vi "sendFloat32.vi"() -> ()   [LabVIEW 2018, in "LV-Julia_ZMQ-Roundtrip_lib.lvlib"]
uses:
  LV-Julia_ZMQ-Roundtrip_lib.lvlib
  Julia functions enum.ctl
  example args cluster.ctl
  example server response cluster.ctl
  Commands v2.ctl
  Server or client state.ctl
  commands LV2Jl.ctl
  5d385633-7562-4640-8300-e9530f023818.vi
  fc45eb44-e6a9-447c-a7e0-b6aef0924f0a.vi
  9ad41121-06aa-4420-b411-b77d699816f6.vi
  cb7a600e-1a3f-45a0-9149-1773accb9ab7.vi
  fc45eb44-e6a9-447c-a7e0-b6aef0924f0a.vi/4c353dce-99c3-41b4-b8c4-9908892ab143.vi
  9ad41121-06aa-4420-b411-b77d699816f6.vi/58872895-b3b6-45aa-bb43-f7f31652b3d2.vi
  check ID validity.vi
  <vilib>/Utility/error.llb/Error Cluster From Error Code.vi
  convert Jl functions enum to string.vi
panel:
  in  "bytes prepend":i32
  out "parsed response 2":cluster{"nums":dbl[]}
  in  "base":sgl=1.11 format="%#_13g"
  in  "go once":bool
  out "JSON out":string
  out "parsed response":T1 {"bin_lng" format="%.0e"}
  in  "arr size":u32=1 min=1
  out "final error":errorcluster
  out "current error":errorcluster
  out "status":string
  in  "stop":bool
  in  "Arguments":T2={"arg1"=1, "arg2"=3.14}
  in  "fun2call":T3
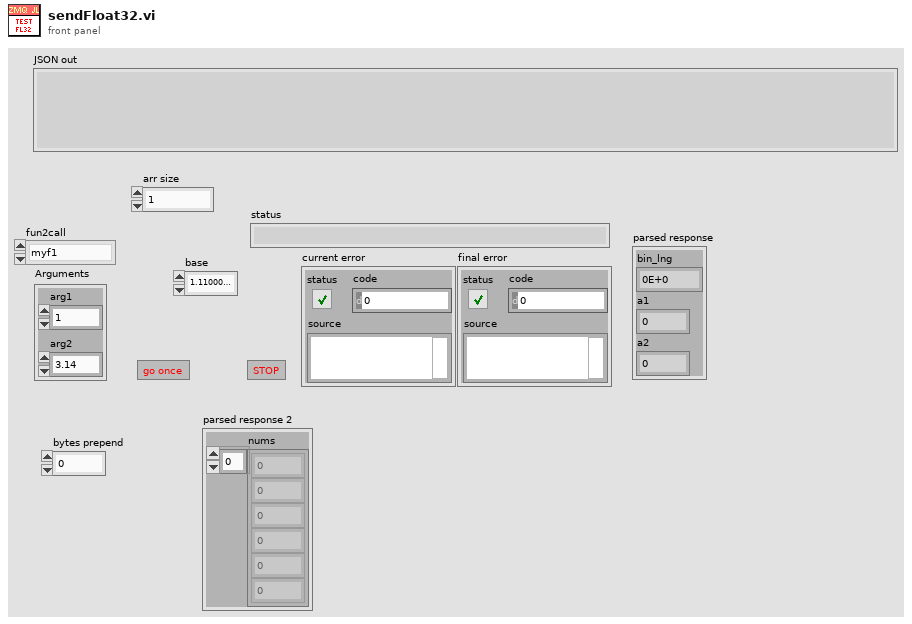
[diagram p1: front panel]
types:
  T1 = typedef "example server response cluster.ctl" = cluster{"bin_lng":i32, "a1":i32, "a2":dbl}
  T2 = typedef "example args cluster.ctl" = cluster{"arg1":i32, "arg2":dbl}
  T3 = typedef "LV-Julia_ZMQ-Roundtrip_lib.lvlib/Julia functions enum.ctl" = enum16{"myf1", "myf2", "myf3", "bin2num"}
  T4 = typedef "LV-Julia_ZMQ-Roundtrip_lib.lvlib/Server or client state.ctl" = enum16{"stopped", "running", "unknown"}
  T5 = typedef "LV-Julia_ZMQ-Roundtrip_lib.lvlib/Commands v2.ctl" = enum16{"Start Jl-server & Init LV-client", "Send request & Get response ", "Stop Jl-server & Cleanup LV-client", "Cleanup LV-client", "Start Jl-server", "Stop Jl-server", "Init LV-Client", "Cleanup LV-Client", "(not allowed)", "Set LV Client state", "Set Jl Server state"}
  T6 = typedef "commands LV2Jl.ctl" = u8
  T7 = cluster{"length":i32, "numtype":string, "start":i32, "dims":i32[], "Tag":string}
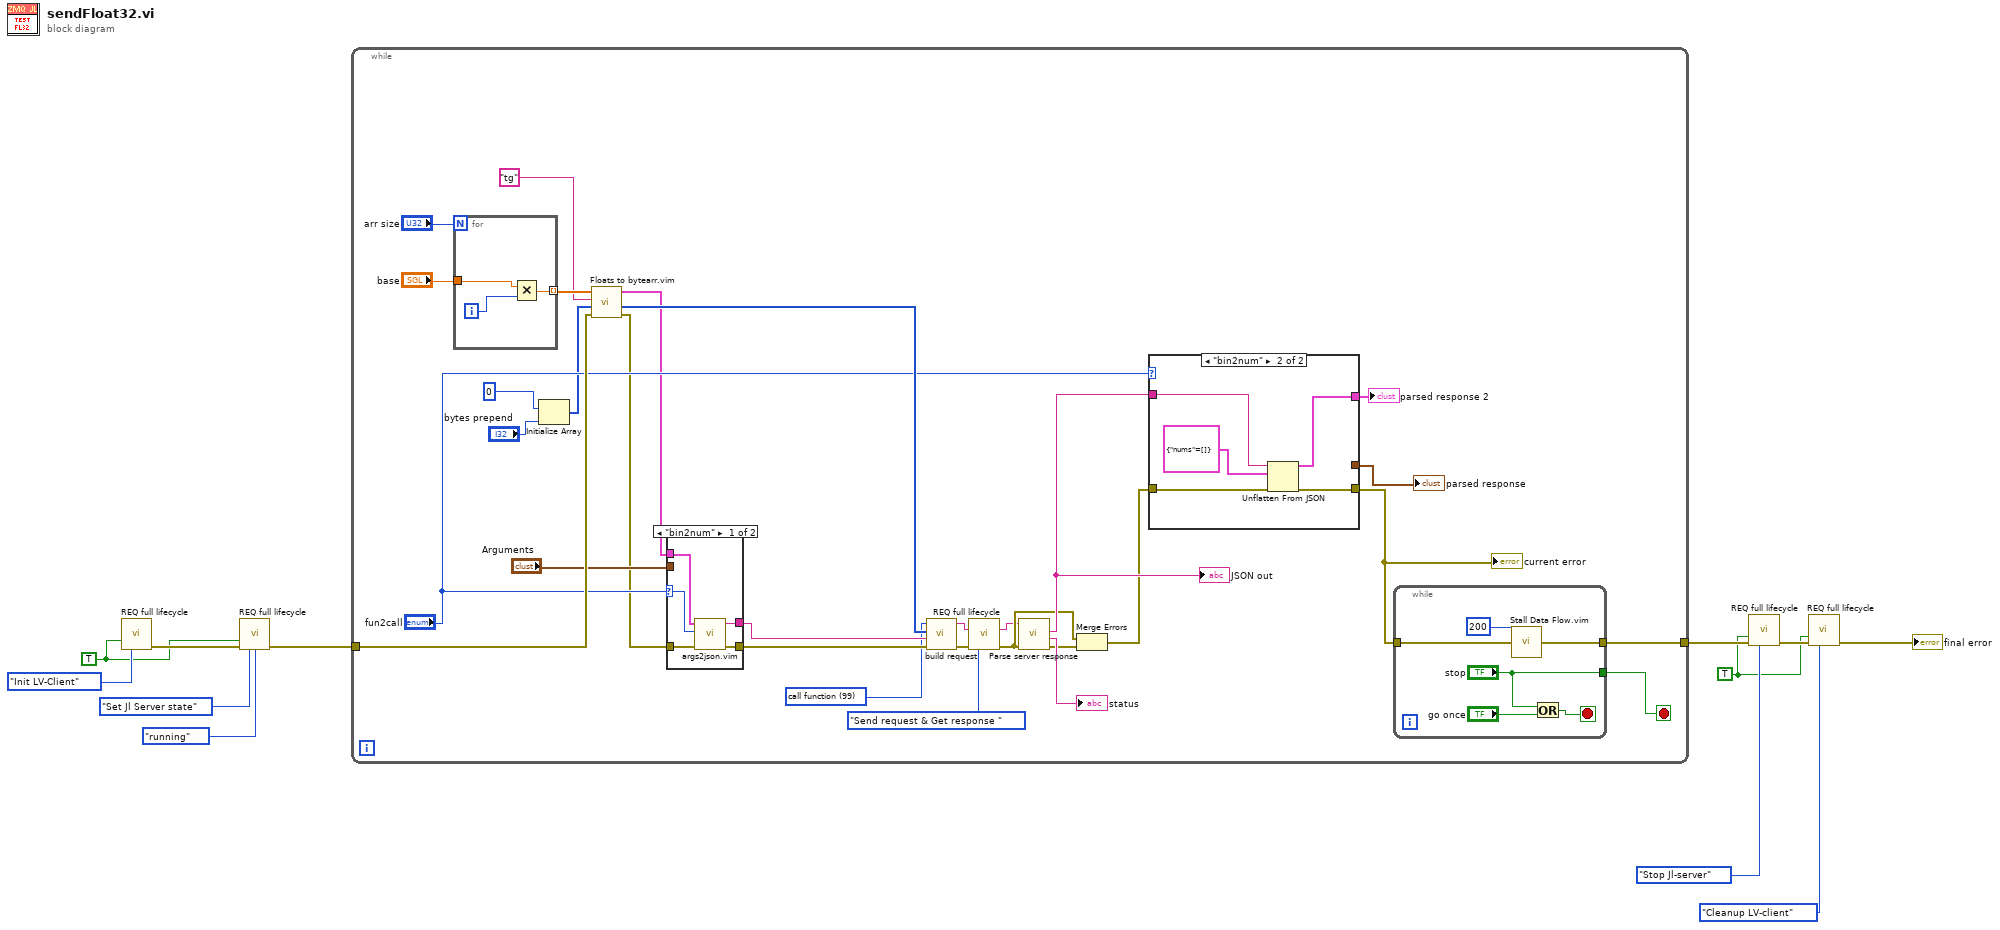
[diagram p0: block diagram]
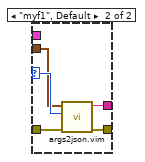
[diagram p2: hidden frame]
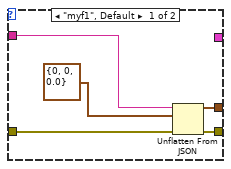
[diagram p3: hidden frame]
diagram:
  w6 = TRUE ("Force command")
  w2 = TRUE ("Force command")
  n1 = call "REQ full lifecycle.vi"("Force command"=w2, "command"=Commands_v2."Init LV-Client") -> ("error out"=w5:errorcluster)  [unwired: 10 in, 3 out]
  n2 = call "REQ full lifecycle.vi"("Force command"=w2, "error in"=w5, "command"=Commands_v2."Set Jl Server state", "Jl Server state in"=Server_or_client_state."running") -> ("error out"=w4:errorcluster)  [unwired: 8 in, 3 out]
  n3 = while {
    tunnel: w4 -> [w31]
    tunnel: [w29] -> w12
    stop <- w28 stop-if-true
    w22 = T6 99 items=["call function"=99, "ping"=112, "stop"=115] ("Command")
    n4 = for {
      N: "arr size" -> [_]
      tunnel: "base" -> [w55]
      tunnel: [w53] -> w24 mode=indexing
      i -> [w54]
      n5 = Multiply(x=w55, y=w54) -> (x*y=w53:sgl)
    }
    n6 = Initialize Array(u8 0 ("bytes out"), "bytes prepend") -> (w16:u8[])
    n7 = call "Floats to bytearr.vim"("error in (no error)"=w31, 9:w16, "Tag"="tg", "Array in"=w24) -> ("error out"=w13:errorcluster, "bytes out"=w23:u8[], "bindata descr"=w19:T7)  [unwired: 3 in, 2 out]
    n8 = case shown="\"bin2num\"" "fun2call" {
      selector: "fun2call" -> [w43 w49]
      tunnel: [w46 w51] -> w39
      tunnel: [w45 w50] -> w38
      tunnel: w13 -> [w47 w52]
      tunnel: w19 -> [w44 _]
      tunnel: "Arguments" -> [_ w48]
      frame "bin2num" {
        n9 = call "args2json.vim"("error in (no error)"=w47, "fun2call"=w43, "Arguments"=w44) -> ("error out"=w46:errorcluster, "JSON string"=w45:string)  [unwired: 7 in]
      }
      frame "myf1", Default {
        n10 = call "args2json.vim"("error in (no error)"=w52, "fun2call"=w49, "Arguments"=w48) -> ("error out"=w51:errorcluster, "JSON string"=w50:string)  [unwired: 7 in]
      }
    }
    n11 = call "build request.vi"("error in (no error)"=w39, "JSON data"=w38, "binary data"=w23, "Command"=w22) -> ("error out"=w36:errorcluster, "REQ string"=w37:string)  [unwired: 6 in]
    n12 = call "REQ full lifecycle.vi"("data to send"=w37, "error in"=w36, "command"=Commands_v2."Send request & Get response ") -> ("server response"=w33:string, "error out"=w34:errorcluster)  [unwired: 9 in, 2 out]
    n13 = call "Parse server response.vi"("error in (no error)"=w34, "server response in"=w33) -> ("error out"=w35:errorcluster, "detailed err description"=→"status":string, "JSON out"=w41:string)  [unwired: 3 in, 4 out]
    "JSON out" <- w41
    n14 = Merge Errors(w34, w35) -> (w40:errorcluster)
    n15 = case shown="\"bin2num\"" "fun2call" {
      tunnel: w41 -> [w66 w71]
      tunnel: w40 -> [w65 w70]
      tunnel: [w64 w69] -> w30
      tunnel: [w63 _] -> w27
      tunnel: [_ w67] -> w21
      frame "myf1", Default {
        n16 = Unflatten From JSON(JSON string=w66, type and defaults=T1 {"bin_lng"=0, "a1"=0, "a2"=0.0} ("parsed response"), error in (no error)=w65) -> (value=w63:T1, error out=w64:errorcluster)  [unwired: 4 in]
      }
      frame "bin2num" {
        n17 = Unflatten From JSON(JSON string=w71, type and defaults=cluster{"nums":dbl[]} {"nums"=[]} ("parsed response"), error in (no error)=w70) -> (value=w67:cluster{"nums":dbl[]}, error out=w69:errorcluster)  [unwired: 4 in]
      }
    }
    "current error" <- w30
    "parsed response" <- w27
    "parsed response 2" <- w21
    n18 = while {
      tunnel: w30 -> [w61]
      tunnel: [w60] -> w29
      tunnel: ["stop"] -> w28
      stop <- w57 stop-if-true
      n19 = call "Stall Data Flow.vim"("value in"=w61, "milliseconds to wait"=u32 200) -> ("value out"=w60:errorcluster)  [unwired: 1 out]
      n20 = Or(x="stop", y="go once") -> (x .or. y?=w57:bool)
    }
  }
  n21 = call "REQ full lifecycle.vi"("Force command"=w6, "error in"=w12, "command"=Commands_v2."Stop Jl-server") -> ("error out"=w9:errorcluster)  [unwired: 9 in, 3 out]
  n22 = call "REQ full lifecycle.vi"("Force command"=w6, "error in"=w9, "command"=Commands_v2."Cleanup LV-client") -> ("error out"=→"final error":errorcluster)  [unwired: 9 in, 3 out]
